vi "20201113_wavelength_measurement_both_wedge_with_DFG_i_it_with_arduino.vi"(0 "Session In":T3) -> (4 "vrt. slope":dbl format="%#_9g", 6 "vert intercept":dbl)   [LabVIEW 2021]
uses:
  <vilib>/userDefined/High Color/IMAQdx.ctl
  <vilib>/Analysis/coordinate.llb/2D Cartesian Coordinate Rotation (Array).vi
  <vilib>/Analysis/6fits.llb/Confidence Interval (Linear).vi
  <vilib>/Instr/_visa.llb/VISA Configure Serial Port (Instr).vi
  <vilib>/Analysis/3filter.llb/Zero Phase Filter (DBL).vi
  <vilib>/addons/control/pid/pid.llb/PID (DBL).vi
  <vilib>/Analysis/3filter.llb/Butterworth Filter (DBL).vi
  <vilib>/Utility/file.llb/Write Delimited Spreadsheet (DBL).vi
  <vilib>/vision/driver/NI_Vision_Acquisition_Software.lvlib
  <vilib>/Analysis/NI_AALPro.lvlib
  <vilib>/Analysis/NI_AAL_SigProc.lvlib
  <vilib>/ptbypt/NI_PtbyPt.lvlib
  <resource>/objmgr/imaqdx.rc
  <vilib>/vision/NI_Vision_Development_Module.lvlib
  <vilib>/Analysis/NI_AALBase.lvlib
  <vilib>/addons/control/pid/NI_PID_pid.lvlib
  <vilib>/LabVIEW Interface for Arduino/LabVIEW Interface for Arduino.lvlib
panel:
  out "number 2":dbl
  out "Boolean":bool
  out "initialized array":dbl[](array[numeric])
  out "subarray 2":dbl[](array[numeric])
  out "Array 5":dbl[](array[numeric])
  out "OPO-532":cluster{dbl[], dbl[]}(graph)
  out "x/y":dbl
  out "cm-1":dbl format="%#_12g"
  out "Amplitudes":dbl[](array[numeric])
  in  "threshold 2":dbl format="%0.2f"
  out "output":dbl format="%.2f"
  out "Vertical intercept vs real time":cluster{dbl[], dbl[]}(graph)
  out "Running average 2":dbl
  out "Running average":dbl
  out "Waveform Graph":dbl[](graph)
  out "Waveform Graph 2":dbl[](graph)
  out "Array 4":dbl[](array[numeric])
  out "loop_counter":i32
  out "vert inteer":dbl[](array[numeric])
  in  "dimension size 2":i32=10
  in  "element 2":dbl=0.1 format="%#_15g"
  in  "Slide 2":dbl(slide)=-10.204081632653061
  out "error out 4":errorcluster
  out "Meter":dbl(knob) scale=0.02..0.1 scale format="%#_4g"
  in  "CONTRAST CUTT OFF VALUE":ext=0.015 format="%#_13g"
  out "x-y":ext
  in  "element":dbl=0.1 format="%#_15g"
  in  "dimension size":i32=10
  out "VERT FRINGE":dbl[][](graph)
  in  "Slide":dbl(slide)=-2.6530612244897958
  out "Verticle slope":cluster{dbl[], dbl[]}(graph)
  out "horz intercept value":dbl[](array[numeric])
  out "vert wavelength":cluster{dbl[], dbl[]}(graph)
  out "intercept":dbl
  in  "index 4":i32=30
  in  "vert-vertical_array length":i32=850
  in  "index 3":i32=500
  in  "length 3":i32=1112
  out "horizontal fringe 2":dbl[][](graph)
  in  "length 2":i32=501
  in  "index 2":i32=400
  in  "length":i32=660
  in  "index":i32=90
  out "vert.wl":dbl
  out "d value":dbl format="%#_10e"
  in  "contrast":ext(slide)=0.5 scale=0.0..0.5 scale format="%#_12g"
  in  "order 2":i32=2
  in  "order":i32=1
  in  "thor wedge spacing":dbl=4.997771500000001 step=1e-06 format="%#_13g"
  in  "wedge angle of thor wedge":dbl=0.004681980000000043 format="%#_13g"
  out "second pass wl 2":dbl format="%#_9g"
  in  "horz. fringe width":i32=6 min=3
  out "hor. std dev":dbl format="%0.5f"
  in  "camera property":bool
  in  "saturation":u32(slide) scale=0.0..128.0
  in  "Gain":u32(slide)=1 scale=1.0..128.0
  in  "exposure":ext(slide)=0.5 scale=0.0..0.5 scale format="%#_12g"
  out "EnumStrings[]":string[](array[string])
  out "known wavelength":dbl
  in  "vert width":i32=5 min=3
  out "Locations":dbl[](array[numeric])
  out "x > y?":bool
  out "Buffer Number Out":u32
  out "observed wavelength":dbl
  out "horz.intercept":dbl format="%#_8g"
  out "known wl":dbl[](array[numeric])=[591.188, 591.588, 591.988, 592.388, 592.788, 593.188]
  out "obseved wl":dbl[](array[numeric])=[591.1849, 591.5523, 591.984, 592.366, 592.7809, 593.169]
  out "standard deviation":dbl format="%0.5f"
  out "Loop time (ms) 2":u32
  out "Array 3":ext[](array[numeric])
  out "Array 2":dbl[](array[numeric])
  out "Array":dbl[](array[numeric])
  out "count":dbl
  out "horz.slope":dbl format="%#_7g"
  out "?":string
  out "?":string
  out "initial time":u32
  out "initial array vert":ext[](array[numeric])
  out "Y Resolution":i32
  out "X Resolution":i32
  out "initial array horz":ext[](array[numeric])
  out "initial array vert.  fringe":ext[](array[numeric])
  out "initila array horz. fringe":ext[](array[numeric])
  in  "Tab Control":enum32{"real time wavelength measurement"}(tab)
  out "532 data":bool
  out "OPO data":bool
  in  "?":T1(tab)
  in  "confidence level vert. fringe":dbl=0.65 format="%.2f"
  in  "threshold vert. fringe":dbl=7.0 format="%0.2f"
  in  "sampling freq. vert. fringe":dbl=1.0000000000000002 format="%0.2f"
  in  "calibration factor vert. fringe":dbl=12000.0
  in  "confidence level horz. fringe":dbl=0.65 format="%.2f"
  in  "sampling freq. horz. fringe":dbl=1.0 format="%0.2f"
  in  "threshold horz. fringe":dbl format="%0.2f"
  in  "calibration factor horz. fringe":dbl=1895.0
  out "RAW Image":T2(plugin-control)
  out "vertical Fringes":dbl[](graph)
  out "Horizontal Fringes":dbl[](graph)
  out "Wavelength vs time":cluster{dbl[], dbl[]}[](graph)
  in  "image depth (bits)":string(combo)="8 bit"
  in  "no. of average":i8=1
  in  "millisecond timer value":u16
  in  "sample length":i32=3
  in  "stop":bool
  in  "Calibration":dbl=7.0
  out "second pass wl":dbl format="%#_9g"
  in  "pixel size (nm)":dbl=4500.0 format="%#_13g"
  in  "wedge angle (rad)":dbl=0.008148144500000017 format="%#_13g"
  in  "wedge spacing":dbl=0.8629192 step=1e-06 format="%#_13g"
  out "?":string="wavelength: 632.993 nm"
  out "?":string
  out "?":string
  in  "maximum OPO":dbl=688.7 format="%#_10g"
  in  "minimum 532":dbl=532.2 format="%#_10g"
  in  "minimum OPO":dbl=688.6 format="%#_10g"
  in  "maximum 532":dbl=532.3 format="%#_10g"
  in  "Running average No":i32=7
  out "Running average OPO data":dbl[](graph)
  out "Running average 532 data":dbl[](graph)
  out "horzontal intercept":cluster{dbl[], dbl[]}(graph)
  out "OPO-532":dbl[](graph)
  in  "Feedback sign":i32=-1 format="%2.0f"
  in  "Manual input voltage":dbl format="%_4f"
  in  "setpoint":dbl format="%.7f"
  in  "output range":cluster{"output high":dbl, "output low":dbl}={"output high"=16.0, "output low"=-16.0} {"output low" format="%.2f"; "output high" format="%.2f"}
  out "Output (V)":dbl format="%.2f"
  in  "PID gains":T4={"proportional gain (Kc)"=1.0, "integral time (Ti, min)"=0.001, "derivative time (Td, min)"=0.001} {"derivative time (Td, min)" format="%.3f"; "integral time (Ti, min)" format="%.3f"; "proportional gain (Kc)" format="%.3f"}
  out "Process value":dbl format="%#_8g"
  in  "Feedback ON":bool
  in  "VISA for power supply 2":refnum<visa-resource-name>
  out "read buffer 2":string
  in  "VISA resource":refnum<visa-resource-name>
  in  "Number Of Servos (1)":u8=1
  in  "DIO Pin (2)":u8=2
  out "Angle (Degrees) 3":u8=15
  in  "millisecond multiple 2":u32=15000
  out "Angle (Degrees)":u8=15
  in  "millisecond multiple":u32=15000
  out "Servo motor Current \nAngle (Degrees) 2":u8=15
  in  "stop 2":bool
  in  "Read voltage":bool
  out "error out 2":errorcluster
  out "error out 3":errorcluster
  out "error out":errorcluster
  # "To do:\n\n(1)  Include calibration routine\n(3) Statistics: Std error for last N values (N is user selected) 1st pass\n-> statistics for deviation of intercept (in cm-1 or MHz) last N values"
  # "Control parameter"
  # "First pass cal."
  # "second pass cal."
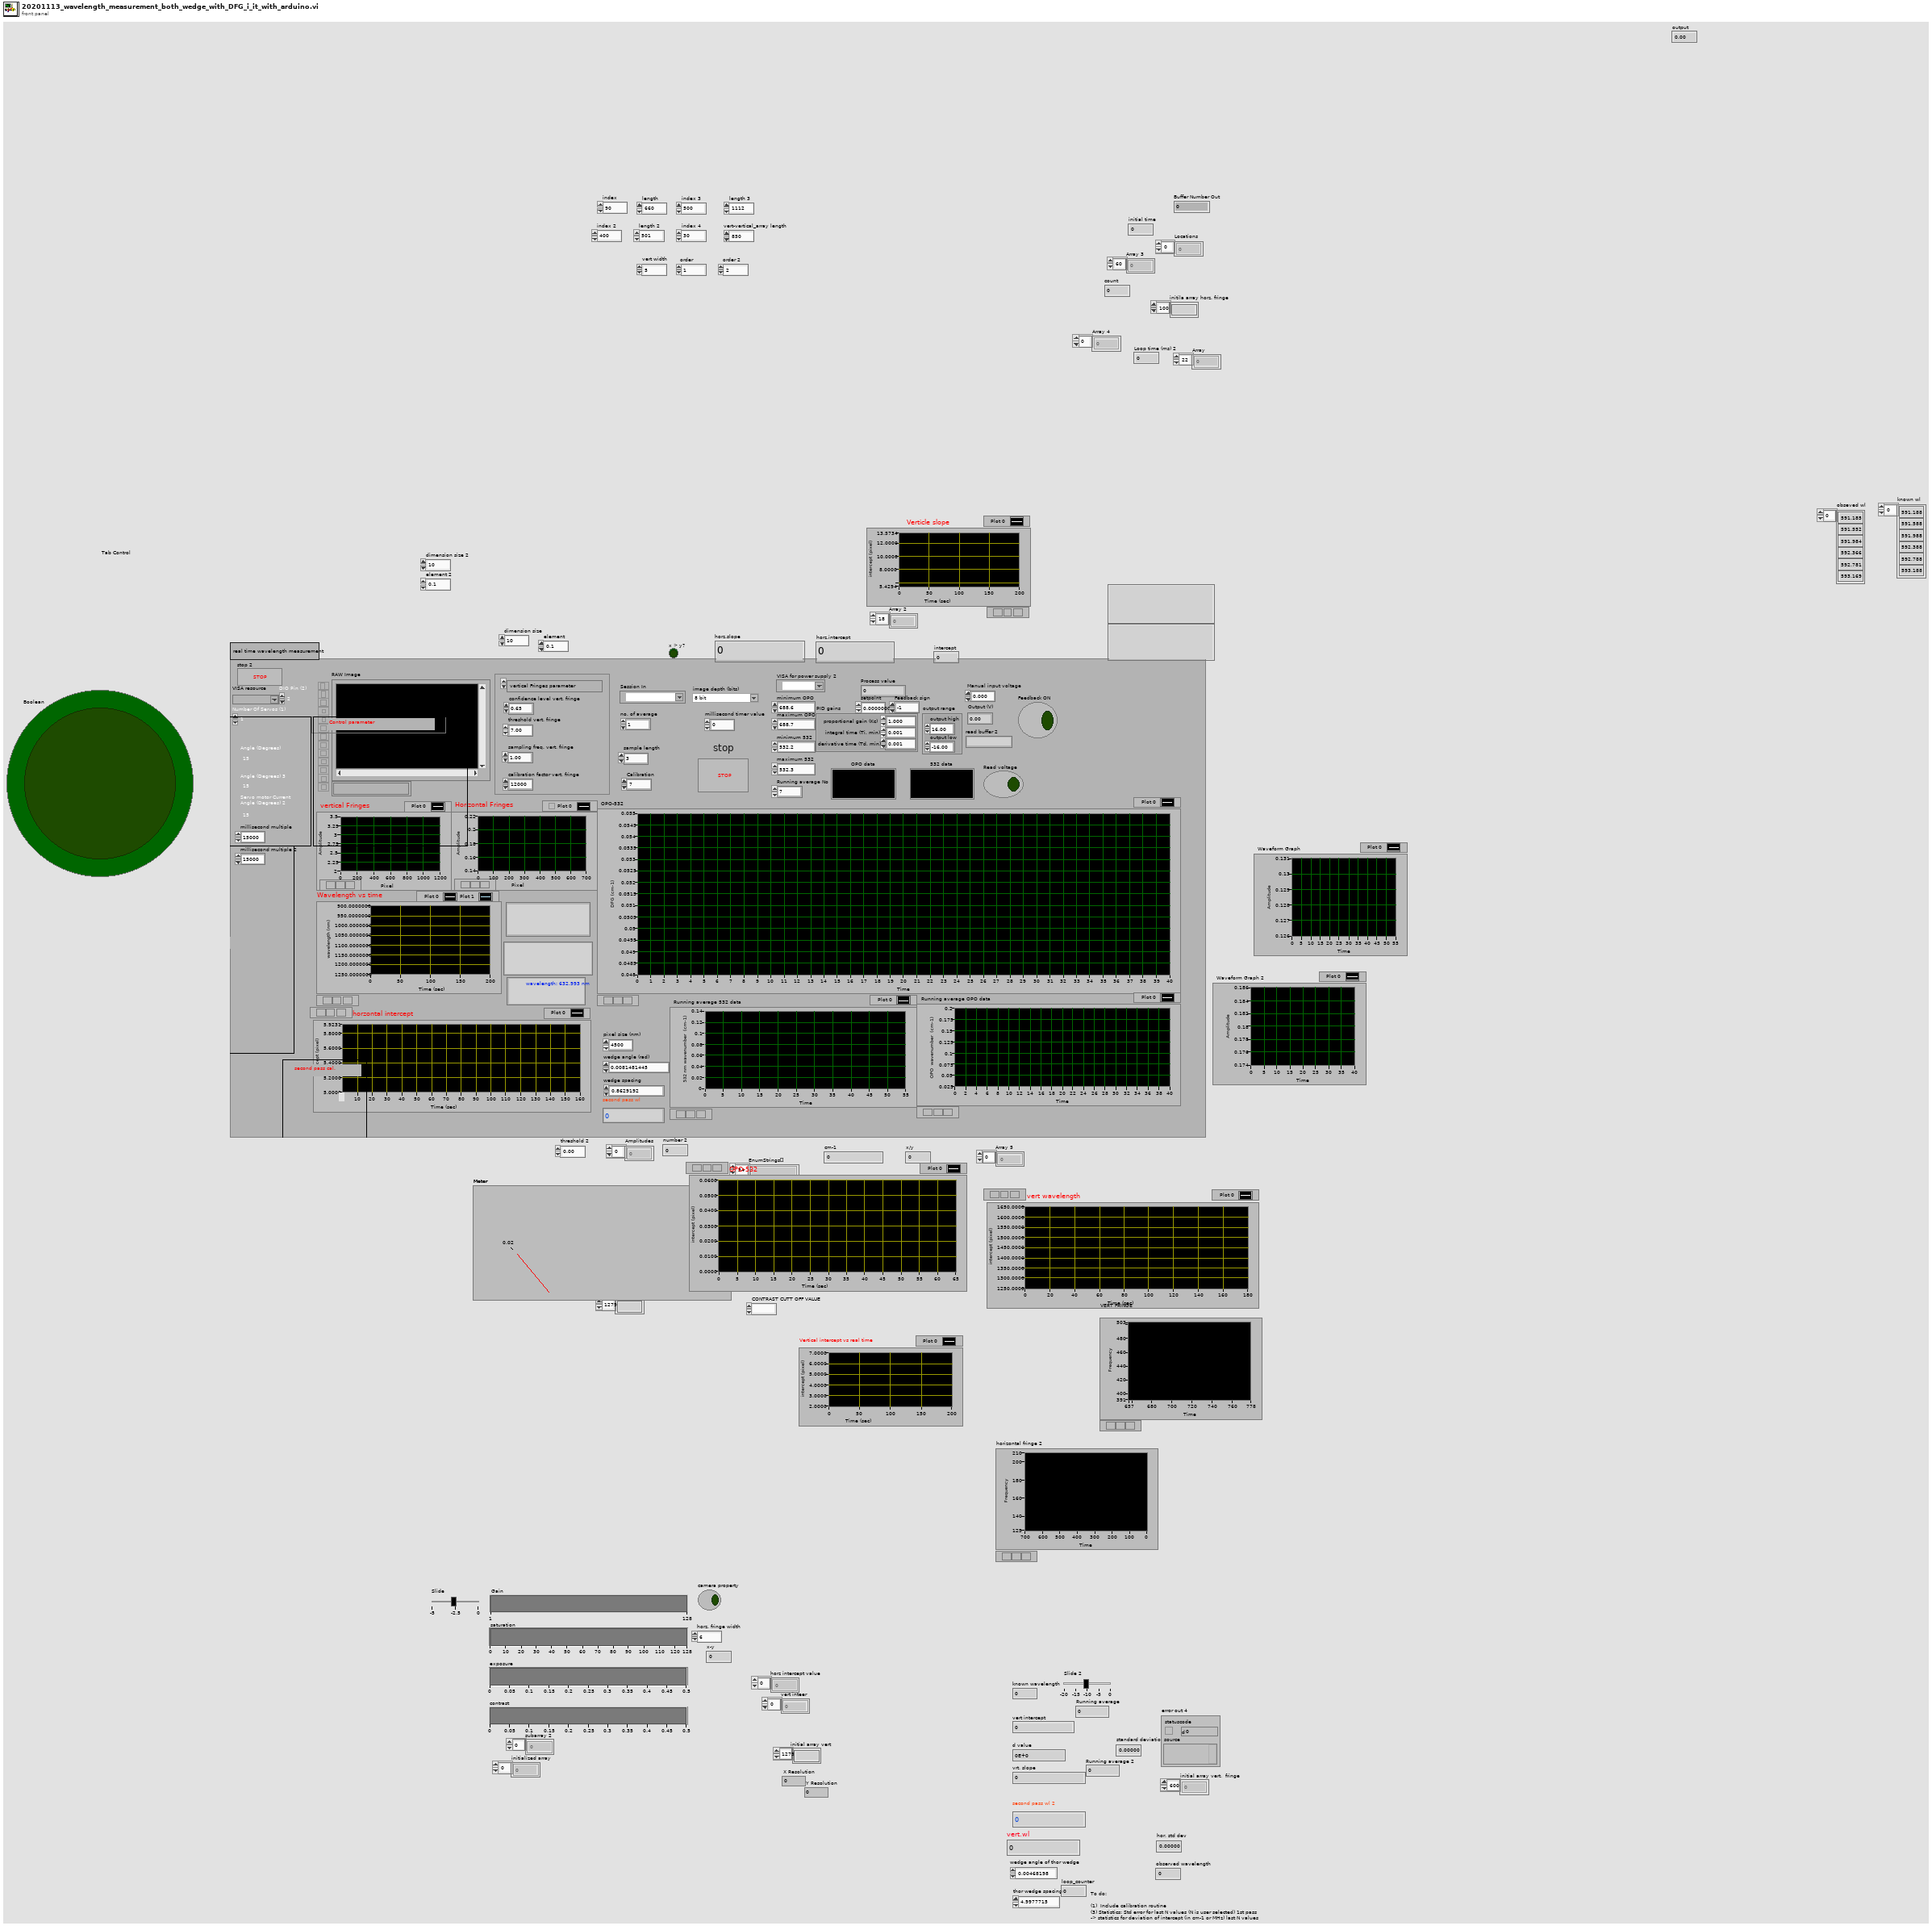
[diagram p1: front panel]
types:
  T1 = enum32{"vertical Fringes parameter", "Horizontal Fringes parameter"}
  T2 = typedef "IMAQ Image.ctl" = refnum<image>
  T3 = typedef "IMAQdx.ctl" = refnum<k21>
  T4 = cluster{"proportional gain (Kc)":dbl, "integral time (Ti, min)":dbl, "derivative time (Td, min)":dbl}
  T5 = typedef "Image Type" = u32
  T6 = typedef "LabVIEW Interface for Arduino.lvlib/Arduino Resource.ctl" = cluster{"VISA resource":refnum<visa-resource-name>, "Board Type":T7, "Connection Type":enum8{"USB / Serial"}, "Bytes Per Packet (15)":u8}
  T7 = typedef "LabVIEW Interface for Arduino.lvlib/Board Type.ctl" = enum16{"Uno", "Dimuelanove w/Atmega 328", "Mega 2560"}
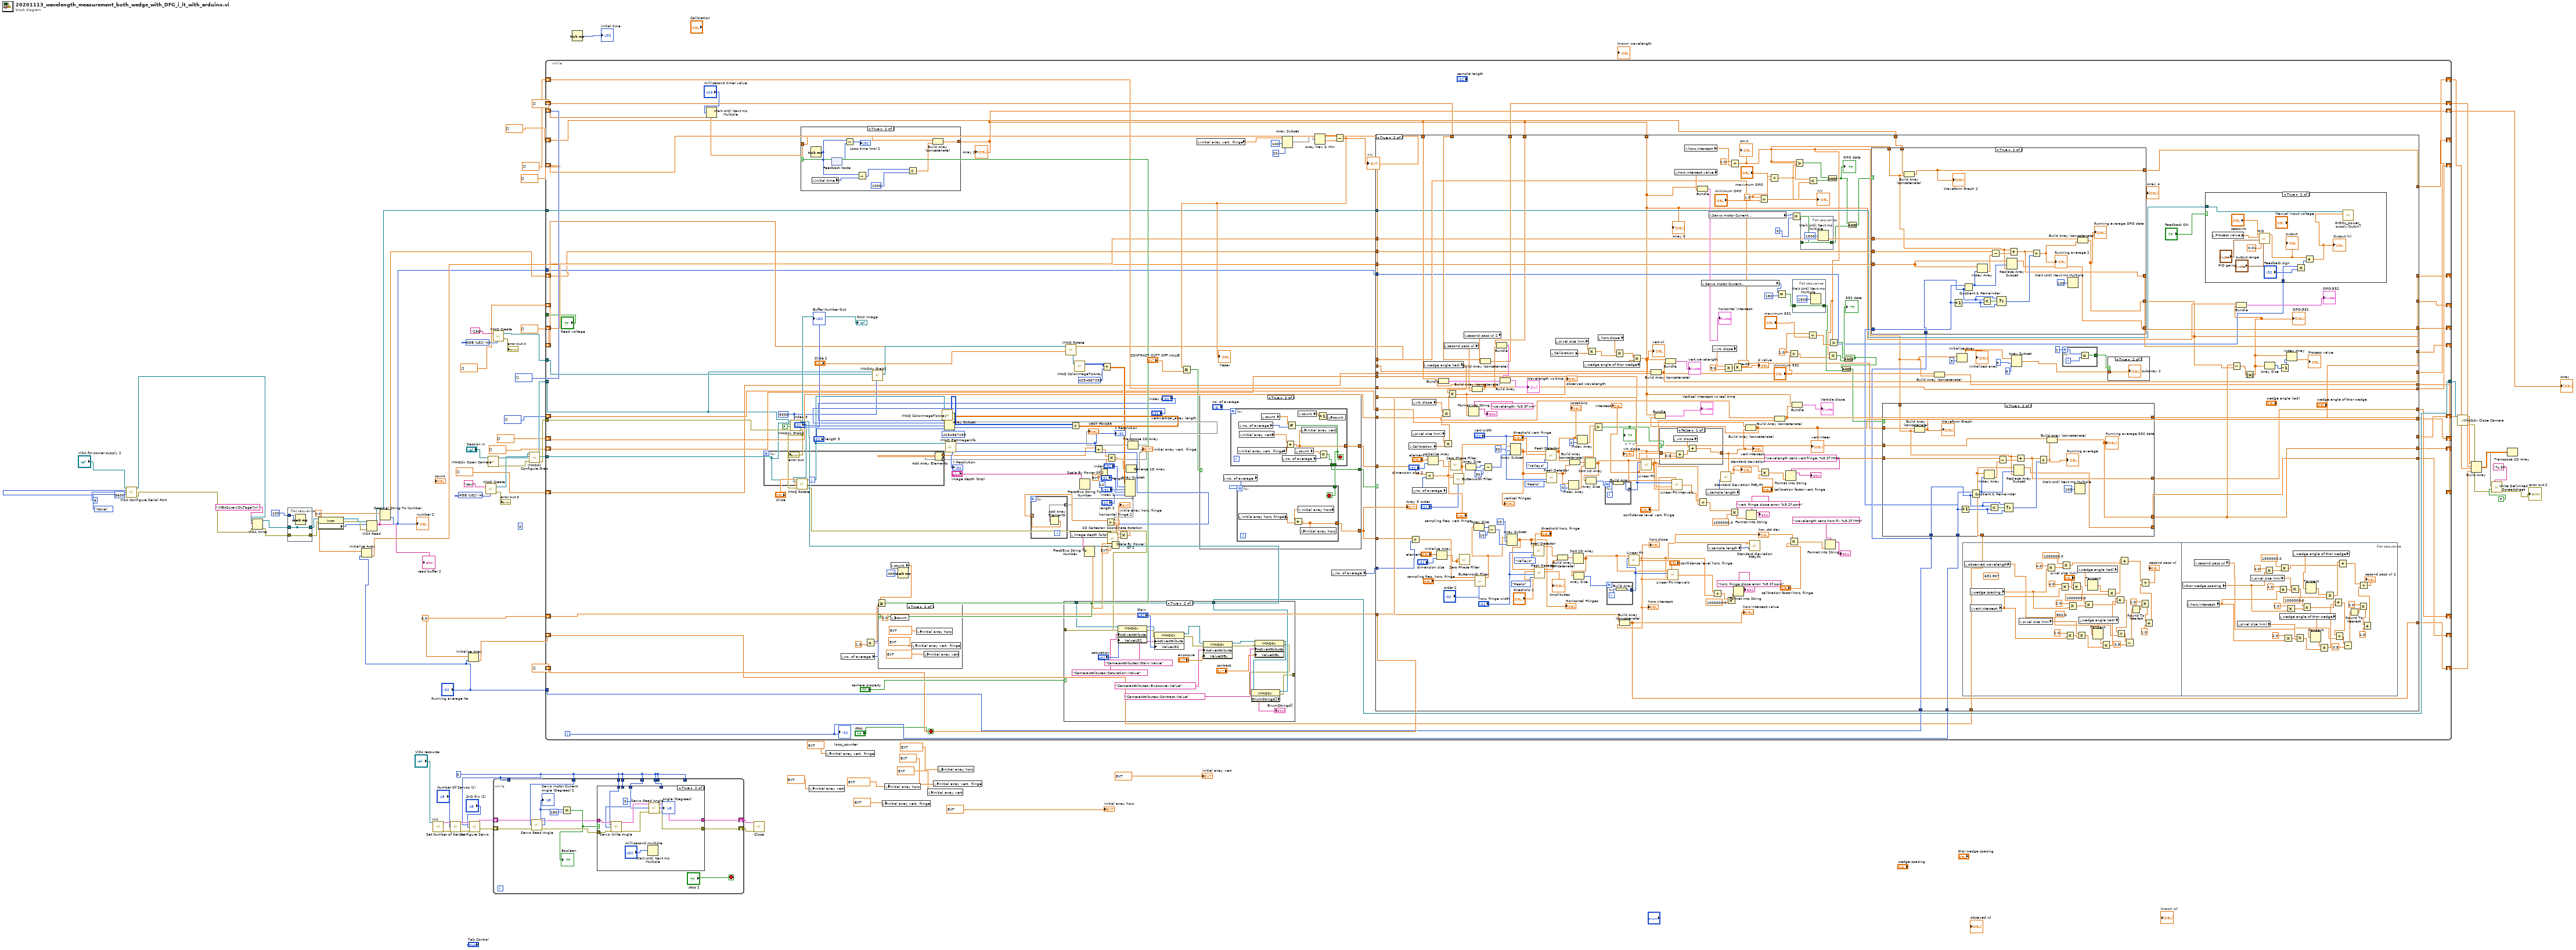
[diagram p0: block diagram]
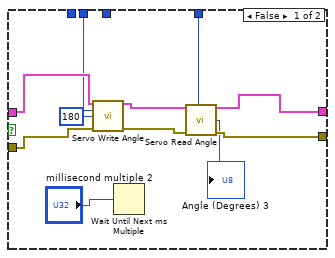
[diagram p2: hidden frame]
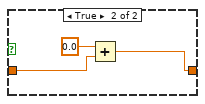
[diagram p12: hidden frame]
diagram:
  w15 = u8 0 ("Servo Number (0)")
  (unwired) u8 0 ("Servo Number (0)")
  w32 = 0.0
  w37 = 0.0
  w54 = T5 4 items=["Grayscale (U8)", "Grayscale (I16)", "Grayscale (SGL)", "Complex (CSG)", "RGB (U32)", "HSL (U32)", "RGB (U64)", "Grayscale (U16)"] ("Image Type")
  w78 = T5 4 items=["Grayscale (U8)", "Grayscale (I16)", "Grayscale (SGL)", "Complex (CSG)", "RGB (U32)", "HSL (U32)", "RGB (U64)", "Grayscale (U16)"] ("Image Type")
  n1 = call-poly "VISA Configure Serial Port"("VISA resource name"="VISA for power supply 2", "baud rate (9600)"=u32 9600, "data bits (8)"=u16 8, "parity (0:none)"=enum16{"None", "Odd", "Even", "Mark", "Space"}."None") -> ("VISA resource name out"=w13:refnum<visa-resource-name>, "error out"=w14:errorcluster)  [unwired: 5 in, 5 out]
  n2 = VISA Write(VISA resource name=w13, write buffer=":MEASure:VOLTage?\n" ("Command"), error in (no error)=w14) -> (VISA resource name out=w11:refnum<visa-resource-name>, error out=w10:errorcluster)  [unwired: 1 out]
  n3 = flat-sequence {
    tunnel: w10 -> [w84]
    tunnel: [w84] -> w8
    tunnel: w11 -> [w83]
    tunnel: [w83] -> _
    tunnel: u32 100 ("delay before read (ms)") -> [w85]
    tunnel: [w83] -> w9
    frame #0 {
      n4 = Wait (ms)(milliseconds to wait=w85) -> ()  [unwired: 1 out]
    }
  }
  n5 = property class="Instr"(reference=w9, error in=w8) -> (reference out=w7:refnum<visa-resource-name>, error out=w6:errorcluster, "Serial Settings:Number of Bytes at Serial Port"=w1:u32)
  n6 = Initialize Array(w32, "Running average No") -> (w33:dbl[])
  n7 = VISA Read(VISA resource name=w7, byte count=w1, error in (no error)=w6) -> (VISA resource name out=w2:refnum<visa-resource-name>, read buffer=w3:string)  [unwired: 2 out]
  "read buffer 2" <- w3
  n8 = Decimal String To Number(string=w3) -> (number=w5:i32)  [unwired: 2 in, 1 out]
  "number 2" <- w5
  n9 = call <vilib>:"Init.vi"("VISA resource"="VISA resource") -> ("Arduino Resource"=w26:T6, "error out"=w25:errorcluster)  [unwired: 17 in]
  n10 = call <vilib>:"Set Number of Servos.vi"("Arduino Resource"=w26, "Number Of Servos (1)"="Number Of Servos (1)", "error in"=w25) -> ("Arduino Resource"=w21:T6, "error out"=w20:errorcluster)  [unwired: 11 in]
  n11 = Initialize Array(w37, "Running average No") -> (w38:dbl[])
  n12 = call <vilib>:"Configure Servo.vi"("Arduino Resource"=w21, "Servo Number (0)"=w15, "DIO Pin (2)"="DIO Pin (2)", "error in"=w20) -> ("Arduino Resource"=w19:T6, "error out"=w18:errorcluster)  [unwired: 10 in]
  n13 = call "IMAQ Create"("Image Name"="sau", "Image Type"=w78) -> ("New Image"=w76:T2, "error out"=→"error out 3":errorcluster)  [unwired: 3 in]
  n14 = call <vilib>:"IMAQdx Open Camera.vi"("Session In"="Session In") -> ("error out"=w56:errorcluster, "Session Out"=w55:T3)  [unwired: 9 in]
  n15 = call "IMAQ Create"("Image Name"="256", "Image Type"=w54) -> ("New Image"=w51:T2, "error out"=→"error out 4":errorcluster)  [unwired: 3 in]
  n16 = while {
    tunnel: w15 -> [w100]
    shift-right: [w94] -> w24
    shift-left: w19 -> [w89]
    shift-right: [w93] -> w23
    shift-left: w18 -> [w88]
    tunnel: w15 -> [_]
    tunnel: w15 -> [_]
    tunnel: w15 -> [w95]
    tunnel: w15 -> [_]
    tunnel: w15 -> [w92]
    tunnel: w15 -> [w91]
    tunnel: w15 -> [w90]
    stop <- "stop 2" stop-if-true
    n17 = call <vilib>:"Servo Read Angle.vi"("Arduino Resource"=w89, "Servo Number"=w100, "error in"=w88) -> ("Arduino Resource"=w97:T6, "Angle (Degrees)"=w99:u8, "error out"=w96:errorcluster)  [unwired: 10 in]
    "Servo motor Current \nAngle (Degrees) 2" <- w99
    n18 = Equal?(x=w99, y=u8 180) -> (x = y?=w87:bool)
    "Boolean" <- w87
    n19 = case shown="True" w87 {
      tunnel: w97 -> [w109 w122]
      tunnel: w96 -> [w108 w121]
      tunnel: w95 -> [_ w120]
      tunnel: [w105 w114] -> w94
      tunnel: [w106 w116] -> w93
      tunnel: w92 -> [_ w113]
      tunnel: w91 -> [w104 _]
      tunnel: w90 -> [w103 _]
      frame False {
        n20 = call <vilib>:"Servo Write Angle.vi"("Arduino Resource"=w109, "Servo Number"=w104, "Angle (Degrees)"=u8 180, "error in"=w108) -> ("Arduino Resource"=w110:T6, "error out"=w107:errorcluster)  [unwired: 10 in]
        n21 = Wait Until Next ms Multiple(millisecond multiple="millisecond multiple 2") -> ()  [unwired: 1 out]
        n22 = call <vilib>:"Servo Read Angle.vi"("Arduino Resource"=w110, "Servo Number"=w103, "error in"=w107) -> ("Arduino Resource"=w105:T6, "Angle (Degrees)"=→"Angle (Degrees) 3":u8, "error out"=w106:errorcluster)  [unwired: 10 in]
      }
      frame True {
        n23 = call <vilib>:"Servo Write Angle.vi"("Arduino Resource"=w122, "Servo Number"=w120, "Angle (Degrees)"=u8 0, "error in"=w121) -> ("Arduino Resource"=w115:T6, "error out"=w117:errorcluster)  [unwired: 10 in]
        n24 = Wait Until Next ms Multiple(millisecond multiple="millisecond multiple") -> ()  [unwired: 1 out]
        n25 = call <vilib>:"Servo Read Angle.vi"("Arduino Resource"=w115, "Servo Number"=w113, "error in"=w117) -> ("Arduino Resource"=w114:T6, "Angle (Degrees)"=→"Angle (Degrees)":u8, "error out"=w116:errorcluster)  [unwired: 10 in]
      }
    }
  }
  n26 = call <vilib>:"IMAQdx Configure Grab.vi"("error in"=w56, "Session In"=w55) -> ("error out"=w75:errorcluster, "Session Out"=w81:T3)  [unwired: 8 in]
  n27 = while {
    tunnel: w75 -> [w232]
    tunnel: w76 -> [w167]
    tunnel: w81 -> [w127]
    tunnel: [w201] -> w72
    shift-right: [w203] -> w48
    shift-left: i32[] [] -> [w225]
    shift-right: [w210] -> w41
    shift-left: dbl[] [] -> [w205]
    shift-right: [w197] -> w61
    shift-left: u32[] [] -> [w211]
    shift-right: [w198] -> w47
    shift-left: dbl[] [] -> [w199]
    shift-right: [w186] -> w46
    shift-left: dbl[] [] -> [w185]
    shift-right: [w183] -> _
    shift-left: dbl[] [] -> [w182]
    shift-right: [w150] -> _
    shift-left: dbl[] [] -> [w179]
    tunnel: w51 -> [w128]
    shift-right: [w148] -> _
    shift-left: dbl[] [] -> [w147]
    shift-right: [w146] -> _
    shift-left: dbl[] [] -> [w145]
    tunnel: "Running average No" -> [w143]
    shift-right: [w142] -> _
    shift-left: w38 -> [w141]
    shift-right: [w140] -> _
    shift-left: w37 -> [w139]
    shift-right: [w137] -> _
    shift-left: dbl[] [] -> [w138]
    shift-right: [w133] -> _
    shift-left: dbl[] [] -> [w136]
    shift-right: [w135] -> _
    shift-left: w33 -> [w134]
    shift-right: [w132] -> _
    shift-left: w32 -> [w131]
    shift-right: [w130] -> _
    shift-left: dbl[] [] -> [w129]
    tunnel: ["Read voltage"] -> _
    tunnel: w5 -> [w124]
    tunnel: w2 -> [w123]
    i -> [w144]
    stop <- "stop" stop-if-true
    w157 = 5000 ("Timeout (ms)")
    n28 = Wait Until Next ms Multiple(millisecond multiple="millisecond timer value") -> ()  [unwired: 1 out]
    n29 = call <vilib>:"IMAQdx Grab2.vi"("Timeout (ms)"=w157, "error in"=w232, "Wait for Next Buffer? (Yes)"=FALSE, "Image In"=w167, "Session In"=w127) -> ("error out"=w170:errorcluster, "Buffer Number Out"=→"Buffer Number Out":u32, "Image Out"=w168:T2, "Session Out"=w202:T3)  [unwired: 3 in]
    "error out" <- w170
    "RAW Image" <- w168
    n30 = call "IMAQ Rotate"("error in (no error)"=w170, "Angle (degrees)"="Slide", "Image Dst"=w168, "Image Src"=w167) -> ("error out"=w169:errorcluster, "Image Dst Out"=w171:T2)  [unwired: 6 in]
    n31 = local read "no. of average"() -> (w214:i8)
    n32 = Add(x=w214, y=1.0) -> (x+y=w213:dbl)
    n33 = call <vilib>:"IMAQdx Grab2.vi"("Timeout (ms)"=w157, "Image In"=w128, "Session In"=w127) -> ("Image Out"=w152:T2)  [unwired: 5 in, 3 out]
    n34 = local read "count"() -> (w216:dbl)
    n35 = Greater Or Equal?(x=w216, y=w213) -> (x >= y?=w212:bool)
    n36 = case shown="True" w212 {
      tunnel: [w277 w280] -> w197
      tunnel: w211 -> [w277 w278]
      frame False {
      }
      frame True {
        n37 = Tick Count (ms)() -> (millisecond timer value=w281:u32)
        n38 = local read "initial time"() -> (w285:u32)
        n39 = feedback #1() -> (w286:u32)  [unwired: 1 in]
        n40 = feedback-in #1(w281) -> ()
        n41 = Subtract(x=w281, y=w286) -> (x-y=→"Loop time (ms) 2":u32)
        n42 = Subtract(x=w281, y=w285) -> (x-y=w282:u32)
        n43 = Divide(x=w282, y=1000) -> (x/y=w279:dbl)
        n44 = Build Array (concatenate)(w278, w279) -> (w280:dbl[])
      }
    }
    "Array 2" <- w197
    n45 = case shown="True" w212 {
      frame False {
      }
      frame True {
        n46 = local write "count"(0.0 ("count")) -> ()
        n47 = local write "initial array vert.  fringe"(ext[] array[1280 elements] ("initial array")) -> ()
        n48 = local write "initial array horz"(ext[] array[1280 elements] ("initial array 2")) -> ()
        n49 = local write "initial array vert"(ext[] array[1282 elements] ("initial array vert")) -> ()
      }
    }
    n50 = Wait (ms)(milliseconds to wait=u32 400) -> ()  [unwired: 1 out]
    n51 = call "IMAQ ColorImageToArray"("Image"=w171) -> ("Image Pixels (U32)"=w229:u32[][])  [unwired: 3 in, 2 out]
    n52 = call "IMAQ GetImageInfo"("Image"=w171) -> ("Y Resolution"=w227:i32, "X Resolution"=w226:i32)  [unwired: 3 in, 6 out]
    "Y Resolution" <- w227
    "X Resolution" <- w226
    n53 = case shown="True" "camera property" {
      tunnel: w169 -> [w254 w256]
      tunnel: w202 -> [w255 w257]
      tunnel: [w255 w266] -> w201
      tunnel: [w254 w264] -> _
      frame False {
      }
      frame True {
        n54 = property class="IMAQdx"(reference=w257, error in=w256, "ActiveAttribute"="CameraAttributes::Saturation::Value", "ValueU32"="saturation") -> (reference out=w269:T3, error out=w270:errorcluster)
        n55 = property class="IMAQdx"(reference=w269, error in=w270, "ActiveAttribute"="CameraAttributes::Gain::Value", "ValueU32"="Gain") -> (reference out=w274:T3, error out=w273:errorcluster)
        n56 = property class="IMAQdx"(reference=w274, error in=w273, "ActiveAttribute"="CameraAttributes::Exposure::Value", "ValueDBL"="exposure") -> (reference out=w263:T3, error out=w259:errorcluster)
        n57 = property class="IMAQdx"(reference=w263, error in=w259, "ActiveAttribute"="CameraAttributes::Contrast::Value", "ValueDBL"="contrast") -> (reference out=w262:T3, error out=w258:errorcluster)
        n58 = property class="IMAQdx"(reference=w262, error in=w258) -> (reference out=w266:T3, error out=w264:errorcluster, "EnumStrings[]"=→"EnumStrings[]":string[])
      }
    }
    n59 = call "IMAQ Rotate"("Angle (degrees)"="Slide 2", "Image Src"=w152) -> ("Image Dst Out"=w151:T2)  [unwired: 8 in, 1 out]
    n60 = Divide(x=w229, y=u32 4294967295) -> (x/y=w180:dbl[][])
    n61 = Array Subset(array=w180, index (row)="index 4", length (row)="vert-vertical_array length", index (col)="index 3", length (col)="length 3") -> (w188:dbl[][])
    n62 = local read "image depth (bits)"() -> (w206:string)
    n63 = call "IMAQ ColorImageToArray"("Image"=w151) -> ("Image Pixels (U32)"=w156:u32[][])  [unwired: 3 in, 2 out]
    n64 = Fract/Exp String To Number(string="image depth (bits)") -> ()  [unwired: 3 in, 2 out]
    n65 = Fract/Exp String To Number(string=w206) -> (number=w207:dbl)  [unwired: 3 in, 1 out]
    n66 = Scale By Power Of 2(n=i16 12, x=ext 1.0) -> (x*2^n=w221:ext)
    n67 = Divide(x=w156, y=u32 4294967295) -> (x/y=w154:dbl[][])
    n68 = call-poly <vilib>:"2D Cartesian Coordinate Rotation.vi"() -> ()  [unwired: 9 in, 3 out]
    n69 = Scale By Power Of 2(n=w207, x=ext 1.0) -> (x*2^n=w217:ext)
    n70 = Array Subset(array=w154, index (row)="index", length (row)="length", index (col)="index 2", length (col)="length 2") -> (w193:dbl[][])
    "horizontal fringe 2" <- w193
    n71 = for {
      tunnel: [w653] -> w220 mode=indexing
      tunnel: w193 -> [w652] mode=indexing
      n72 = Add Array Elements(numeric array=w652) -> (sum=w653:dbl)
    }
    n73 = Divide(x=w220, y=w226) -> (x/y=w219:dbl[])
    n74 = Multiply(x=w219, y=w217) -> (x*y=→"initila array horz. fringe":ext[])
    n75 = Transpose 2D Array(2D array=w188) -> (transposed array=w166:dbl[][])
    "VERT FRINGE" <- w166
    n76 = for {
      tunnel: [w655] -> w224 mode=indexing
      tunnel: w166 -> [w654] mode=indexing
      n77 = Add Array Elements(numeric array=w654) -> (sum=w655:dbl)
    }
    n78 = Divide(x=w224, y=w227) -> (x/y=w223:dbl[])
    n79 = Multiply(x=w223, y=w221) -> (x*y=w187:ext[])
    n80 = Reverse 1D Array(array=w187) -> (reversed array=→"initial array vert.  fringe":ext[])
    n81 = local read "initial array vert.  fringe"() -> (w164:ext[])
    n82 = Array Subset(array=w164, index=100, length=20) -> (w163:ext[])
    n83 = Array Max & Min(array=w163) -> (max value=w162:ext, min value=w161:ext)  [unwired: 2 out]
    n84 = local read "no. of average"() -> (w209:i8)
    n85 = Subtract(x=w162, y=w161) -> (x-y=w158:ext)
    "x-y" <- w158
    "Meter" <- w158
    n86 = Greater Or Equal?(x=w158, y="CONTRAST CUTT OFF VALUE") -> (x >= y?=w160:bool)
    n87 = case shown="True" w160 {
      tunnel: [_ w235] -> w177
      tunnel: [_ w234] -> w175
      tunnel: [_ w233] -> w165
      frame False {
      }
      frame True {
        n88 = local read "no. of average"() -> (w237:i8)
        n89 = for {
          N: "no. of average" -> [_]
          tunnel: [w251] -> w235
          tunnel: [w246] -> w233
          tunnel: [w243] -> w236
          stop <- w243 stop-if-true
          n90 = local read "initial array vert.  fringe"() -> (w253:ext[])
          n91 = local read "no. of average"() -> (w244:i8)
          n92 = local read "initial array vert"() -> (w252:ext[])
          n93 = local read "count"() -> (w245:dbl)
          n94 = local read "no. of average"() -> (w250:i8)
          n95 = Add(x=w252, y=w253) -> (x+y=w251:ext[])
          n96 = Not Equal?(x=w245, y=w244) -> (x != y?=w243:bool)
          n97 = local read "count"() -> (w249:dbl)
          n98 = local read "count"() -> (w248:dbl)
          n99 = local write "initial array vert"(w251) -> ()
          n100 = Increment(x=w248) -> (x+1=w247:dbl)
          n101 = Equal?(x=w249, y=w250) -> (x = y?=w246:bool)
          n102 = local write "count"(w247) -> ()
        }
        n103 = for {
          N: w237 -> [_]
          tunnel: [w242] -> w234
          tunnel: w236 -> [w239]
          stop <- w239 stop-if-true
          n104 = local read "initila array horz. fringe"() -> (w240:ext[])
          n105 = local read "initial array horz"() -> (w241:ext[])
          n106 = Add(x=w241, y=w240) -> (x+y=w242:ext[])
          n107 = local write "initial array horz"(w242) -> ()
        }
      }
    }
    "Array 3" <- w175
    n108 = case shown="True" w165 {
      tunnel: [w304 w475] -> w203
      tunnel: w225 -> [w304 w502]
      tunnel: w175 -> [_ w500]
      tunnel: w177 -> [_ w499]
      tunnel: w197 -> [_ w480]
      tunnel: [w305 w330] -> w210
      tunnel: w197 -> [_ w332]
      tunnel: w209 -> [_ w479]
      tunnel: w205 -> [w305 w476]
      tunnel: [w303 w421] -> w198
      tunnel: w199 -> [w303 w423]
      tunnel: w197 -> [_ w422]
      tunnel: [w302 w399] -> w186
      tunnel: w185 -> [w302 w400]
      tunnel: w182 -> [w301 w397]
      tunnel: [w301 w396] -> w183
      tunnel: w179 -> [w300 w393]
      tunnel: [w300 w390] -> w150
      tunnel: w147 -> [w299 w373]
      tunnel: [w299 w374] -> w148
      tunnel: [w298 w367] -> w146
      tunnel: w145 -> [w298 w368]
      tunnel: w144 -> [_ w358]
      tunnel: w143 -> [_ w359]
      tunnel: w141 -> [w297 w366]
      tunnel: [w297 w365] -> w142
      tunnel: [w296 w364] -> w140
      tunnel: w139 -> [w296 w363]
      tunnel: w138 -> [w295 w362]
      tunnel: [w295 w333] -> w137
      tunnel: w136 -> [w293 w361]
      tunnel: w134 -> [w294 w360]
      tunnel: [w294 w357] -> w135
      tunnel: [w293 w334] -> w133
      tunnel: w131 -> [w292 w356]
      tunnel: [w292 w355] -> w132
      tunnel: w123 -> [_ w353]
      tunnel: w124 -> [_ w352]
      tunnel: w129 -> [w291 w329]
      tunnel: [w291 w321] -> w130
      frame False {
      }
      frame True {
        w337 = 1.0 ("x")
        w342 = 1.0 ("x")
        n109 = local read "Calibration"() -> (w442:dbl)
        n110 = Divide(x=w500, y=w479) -> (x/y=w381:ext[])
        n111 = local read "pixel size (nm)"() -> (w440:dbl)
        n112 = local read "vrt. slope"() -> (w447:dbl)
        n113 = local read "no. of average"() -> (w501:i8)
        n114 = local read "wedge angle (rad)"() -> (w443:dbl)
        n115 = Divide(x=w499, y=w501) -> (x/y=w384:ext[])
        n116 = Initialize Array("element 2", "dimension size 2") -> (w387:dbl[])
        n117 = Initialize Array("element", "dimension size") -> (w383:dbl[])
        n118 = Multiply(x=w440, y=w442) -> (x*y=w441:dbl)
        n119 = Multiply(x=w447, y=w441) -> (x*y=w446:dbl)
        n120 = local read "second pass wl"() -> (w445:dbl)
        n121 = Multiply(x=w443, y=w446) -> (x*y=w444:dbl)
        "observed wavelength" <- w444
        n122 = call-poly <vilib>:"Zero Phase Filter.vi"("Forward Coefficients"=w387, "X"=w384) -> ()  [unwired: 8 in, 2 out]
        n123 = call-poly <vilib>:"Butterworth Filter.vi"("order"="order", "sampling freq: fs"="sampling freq. vert. fringe", "X"=w384) -> ("Filtered X"=w382:dbl[])  [unwired: 5 in, 1 out]
        n124 = call-poly <vilib>:"Zero Phase Filter.vi"("Forward Coefficients"=w383, "Reverse Coefficients"=w383) -> ()  [unwired: 8 in, 2 out]
        n125 = local read "second pass wl 2"() -> (w424:dbl)
        n126 = Array Size(array=w382) -> (size(s)=w428:i32)
        n127 = Format Into String(format string="wavelength: %5.3f nm", w444) -> (resulting string=→"?":string)  [unwired: 2 in, 1 out]
        n128 = Build Array (concatenate)(w476, w445) -> (w330:dbl[])
        n129 = Bundle(w480, w330) -> (w419:cluster{dbl[], dbl[]})  [unwired: 1 in]
        n130 = call-poly <vilib>:"Butterworth Filter.vi"("order"="order 2", "sampling freq: fs"="sampling freq. horz. fringe", "X"=w381) -> ("Filtered X"=w380:dbl[])  [unwired: 5 in, 1 out]
        n131 = Array Size(array=w380) -> (size(s)=w431:i32)
        n132 = Build Array (concatenate)(w423, w424) -> (w421:dbl[])
        n133 = Subtract(x=w428, y=50) -> (x-y=w426:i32)
        n134 = Subtract(x=w431, y=10) -> (x-y=w430:i32)
        n135 = Bundle(w422, w330) -> (w420:cluster{dbl[], dbl[]})  [unwired: 1 in]
        n136 = Build Array(w420, w419) -> (→"Wavelength vs time":cluster{dbl[], dbl[]}[])
        n137 = Array Subset(array=w380, index=10, length=w430) -> (w412:dbl[])
        "Horizontal Fringes" <- w412
        n138 = Array Subset(array=w382, index=30, length=w426) -> (w402:dbl[])
        "vertical Fringes" <- w402
        n139 = call <vilib>:"Peak Detector.vi"("peaks/valleys"=enum32{"Peaks", "Valleys"}."Valleys", "width"="horz. fringe width", "threshold"="threshold horz. fringe", "X"=w412) -> ("Locations"=w471:dbl[])  [unwired: 3 in, 4 out]
        n140 = call <vilib>:"Peak Detector.vi"("peaks/valleys"=enum32{"Peaks", "Valleys"}."Peaks", "width"="horz. fringe width", "threshold"="threshold 2", "X"=w412) -> ("Amplitudes"=→"Amplitudes":dbl[], "Locations"=w470:dbl[])  [unwired: 3 in, 3 out]
        n141 = call <vilib>:"Peak Detector.vi"("peaks/valleys"=enum32{"Peaks", "Valleys"}."Valleys", "width"="vert width", "threshold"="threshold vert. fringe", "X"=w402) -> ("Locations"=w457:dbl[])  [unwired: 3 in, 4 out]
        "Locations" <- w457
        n142 = call <vilib>:"Peak Detector.vi"("peaks/valleys"=enum32{"Peaks", "Valleys"}."Peaks", "width"="vert width", "X"=w402) -> ("Locations"=w450:dbl[])  [unwired: 4 in, 4 out]
        n143 = local read "Calibration"() -> (w408:dbl)
        n144 = local read "pixel size (nm)"() -> (w409:dbl)
        n145 = Build Array (concatenate)(w471, w470) -> (w469:dbl[])
        n146 = Index Array(array=w450, index=0) -> (element=w453:dbl)
        n147 = Build Array (concatenate)(w457, w450) -> (w495:dbl[])
        n148 = Sort 1D Array(array=w469) -> (sorted array=w466:dbl[])
        n149 = Array Size(array=w466) -> (size(s)=w468:i32)
        n150 = Index Array(array=w457, index=0) -> (element=w454:dbl)
        n151 = local read "wedge angle of thor wedge"() -> (w404:dbl)
        n152 = Sort 1D Array(array=w495) -> (sorted array=w493:dbl[])
        n153 = Array Size(array=w493) -> (size(s)=w494:i32)
        n154 = Multiply(x=w409, y=w408) -> (x*y=w406:dbl)
        n155 = Greater?(x=w454, y=w453) -> (0:w452:bool)
        "x > y?" <- w452
        n156 = local read "horz.slope"() -> (w407:dbl)
        n157 = for {
          N: w494 -> [_]
          tunnel: [w651] -> w492 mode=concatenating
          i -> [w650]
          n158 = Build Array(w650) -> (w651:i32[])
        }
        n159 = for {
          N: w468 -> [_]
          tunnel: [w577] -> w467 mode=concatenating
          i -> [w576]
          n160 = Build Array(w576) -> (w577:i32[])
        }
        n161 = Multiply(x=w407, y=w406) -> (x*y=w405:dbl)
        n162 = call <vilib>:"Linear Fit.vi"("Y"=w466, "X"=w467) -> ("slope"=w462:dbl, "intercept"=w401:dbl)  [unwired: 9 in, 3 out]
        "horz.slope" <- w462
        "horz.intercept" <- w401
        n163 = Build Array (concatenate)(w400, w401) -> (w399:dbl[])
        "horz intercept value" <- w399
        n164 = Multiply(x=w405, y=w404) -> (x*y=w398:dbl)
        "vert.wl" <- w398
        n165 = call <vilib>:"Linear Fit.vi"("Y"=w493, "X"=w492) -> ("slope"=w392:dbl, "intercept"=w458:dbl)  [unwired: 9 in, 3 out]
        "vrt. slope" <- w392
        "intercept" <- w458
        n166 = Build Array (concatenate)(w397, w398) -> (w396:dbl[])
        n167 = case shown="False" w452 {
          tunnel: w458 -> [w570 w575]
          tunnel: [w572 w574] -> w403
          frame False {
            n168 = local read "vrt. slope"() -> (w571:dbl)
            n169 = Add(x=w570, y=0.0) -> (x+y=w569:dbl)
            n170 = Add(x=w571, y=w569) -> (x+y=w572:dbl)
          }
          frame True {
            n171 = Add(x=0.0, y=w575) -> (x+y=w574:dbl)
          }
        }
        "vert intercept" <- w403
        n172 = Bundle(w332, w396) -> (→"vert wavelength":cluster{dbl[], dbl[]})  [unwired: 1 in]
        n173 = call-poly <vilib>:"Linear Fit Intervals.vi"("Y"=w466, "confidence level"="confidence level horz. fringe", "X"=w467, "slope"=w462, "intercept"=w401) -> ("delta slope"=w434:dbl)  [unwired: 6 in, 4 out]
        n174 = call-poly <vilib>:"Linear Fit Intervals.vi"("Y"=w493, "confidence level"="confidence level vert. fringe", "X"=w492, "slope"=w392, "intercept"=w458) -> ("delta slope"=w488:dbl)  [unwired: 6 in, 4 out]
        n175 = local read "horz intercept value"() -> (w375:dbl[])
        n176 = local read "horz.intercept"() -> (w345:dbl)
        n177 = Bundle(w332, "horz intercept value"=w375) -> (→"horzontal intercept":cluster{dbl[], "horz intercept value":dbl[]})  [unwired: 1 in]
        n178 = Divide(x=w488, y=w392) -> (x/y=w486:dbl)
        n179 = local read "Servo motor Current \nAngle (Degrees) 2"() -> (w316:u8)
        n180 = local read "sample length"() -> (w425:i32)
        n181 = local read "sample length"() -> (w436:i32)
        n182 = local read "Servo motor Current \nAngle (Degrees) 2"() -> (w318:u8)
        n183 = Divide(x=w434, y=w462) -> (x/y=w460:dbl)
        n184 = local read "vrt. slope"() -> (w417:dbl)
        n185 = call <vilib>:"Standard Deviation PtByPt.vi"("x"=w403, "sample length"=w425) -> ("standard deviation"=w481:dbl)  [unwired: 1 in, 2 out]
        "standard deviation" <- w481
        n186 = Multiply(x=w417, y=9.0) -> (x*y=w415:dbl)
        n187 = Multiply(x=w460, y=1000000.0) -> (x*y=w459:dbl)
        n188 = Multiply(x=w486, y=1000000.0) -> (x*y=w485:dbl)
        n189 = Divide(x=1.0, y=w345) -> (x/y=w323:dbl)
        "cm-1" <- w323
        n190 = Multiply(x=w415, y=1e-06) -> (x*y=→"d value":dbl)
        n191 = Format Into String(format string="horz. fringe slope error: %5.2f ppm", w459) -> (resulting string=→"?":string)  [unwired: 2 in, 1 out]
        n192 = Build Array (concatenate)(w502, w403) -> (w475:dbl[])
        "vert inteer" <- w475
        n193 = Bundle(w332, w475) -> (→"Vertical intercept vs real time":cluster{dbl[], dbl[]})  [unwired: 1 in]
        n194 = Format Into String(format string="vert. fringe slope error: %5.2f ppm", w485) -> (resulting string=→"?":string)  [unwired: 2 in, 1 out]
        n195 = call <vilib>:"Standard Deviation PtByPt.vi"("x"=w401, "sample length"=w436) -> ("standard deviation"=w439:dbl)  [unwired: 1 in, 2 out]
        "hor. std dev" <- w439
        n196 = Divide(x=w337, y="minimum OPO") -> (x/y=w338:dbl)
        n197 = Multiply(x=w481, y="calibration factor vert. fringe") -> (x*y=w482:dbl)
        n198 = Divide(x=w337, y="maximum OPO") -> (x/y=w335:dbl)
        "x/y" <- w335
        n199 = Build Array (concatenate)(w393, w392) -> (w390:dbl[])
        n200 = Equal?(x=w316, y=u8 180) -> (x = y?=w314:bool)
        n201 = Format Into String(format string="wavelength sens vert fringe: %5.2f MHz", w482) -> (resulting string=→"?":string)  [unwired: 2 in, 1 out]
        n202 = Divide(x=w342, y="minimum 532") -> (x/y=w343:dbl)
        n203 = Multiply(x=w439, y="calibration factor horz. fringe") -> (x*y=w438:dbl)
        n204 = Equal?(x=w318, y=u8 0) -> (x = y?=w317:bool)
        n205 = Bundle(w332, w390) -> (→"Verticle slope":cluster{dbl[], dbl[]})  [unwired: 1 in]
        n206 = flat-sequence {
          tunnel: [w504] -> w309
          tunnel: w314 -> [w504]
          frame #0 {
            n207 = Wait Until Next ms Multiple(millisecond multiple=u32 1500) -> ()  [unwired: 1 out]
          }
        }
        n208 = Greater?(x=w323, y=w335) -> (0:w371:bool)
        n209 = flat-sequence {
          tunnel: [w506] -> w313
          tunnel: w317 -> [w506]
          frame #0 {
            n210 = Wait Until Next ms Multiple(millisecond multiple=u32 1500) -> ()  [unwired: 1 out]
          }
        }
        n211 = Divide(x=w342, y="maximum 532") -> (x/y=w340:dbl)
        n212 = Less?(x=w323, y=w338) -> (x < y?=w372:bool)
        n213 = Format Into String(format string="wavelength sens horz fri: %5.2f MHz", w438) -> (resulting string=→"?":string)  [unwired: 2 in, 1 out]
        n214 = And(x=w371, y=w372) -> (x .and. y?=w312:bool)
        "OPO data" <- w312
        n215 = Less?(x=w323, y=w343) -> (x < y?=w369:bool)
        n216 = Greater?(x=w323, y=w340) -> (0:w370:bool)
        n217 = And(x=w370, y=w369) -> (x .and. y?=w310:bool)
        "532 data" <- w310
        n218 = And(x=w310, y=w309) -> (x .and. y?=w308:bool)
        n219 = And(x=w312, y=w313) -> (x .and. y?=w311:bool)
        n220 = case shown="True" w311 {
          tunnel: w373 -> [w548 w567]
          tunnel: w323 -> [_ w551]
          tunnel: [w548 w566] -> w374
          tunnel: w361 -> [w546 w557]
          tunnel: w360 -> [w547 w556]
          tunnel: w359 -> [_ w555]
          tunnel: w358 -> [_ w554]
          tunnel: [w547 w553] -> w357
          tunnel: [w546 w552] -> w334
          tunnel: w356 -> [w545 w550]
          tunnel: [w545 w549] -> w355
          frame False {
          }
          frame True {
            n221 = Build Array (concatenate)(w567, w551) -> (w566:dbl[])
            "Waveform Graph 2" <- w566
            n222 = Increment(x=w554) -> (x+1=w558:i32)
            n223 = Quotient & Remainder(x=w554, y=w555) -> (x-y*floor(x/y)=w562:i32)  [unwired: 1 out]
            n224 = Index Array(array=w556, index=w562) -> (element=w564:dbl)
            n225 = Less?(x=w555, y=w558) -> (x < y?=w560:bool)
            n226 = Subtract(x=w550, y=w564) -> (x-y=w563:dbl)
            n227 = Select(t=w555, s=w560, f=w558) -> (s? t:f=w559:i32)
            n228 = Replace Array Subset(array=w556, new element=w551, index=w562) -> (w553:dbl[])
            n229 = Add(x=w551, y=w563) -> (x+y=w549:dbl)
            n230 = Divide(x=w549, y=w559) -> (x/y=w565:dbl)
            "Running average 2" <- w565
            n231 = Wait Until Next ms Multiple(millisecond multiple=u32 100) -> ()  [unwired: 1 out]
            n232 = Build Array (concatenate)(w557, w565) -> (w552:dbl[])
            "Running average OPO data" <- w552
          }
        }
        n233 = case shown="True" w308 {
          tunnel: w368 -> [w525 w543]
          tunnel: w323 -> [_ w535]
          tunnel: [w525 w544] -> w367
          tunnel: w358 -> [_ w534]
          tunnel: w359 -> [_ w533]
          tunnel: w366 -> [w524 w532]
          tunnel: [w524 w531] -> w365
          tunnel: [w523 w530] -> w364
          tunnel: w363 -> [w523 w529]
          tunnel: w362 -> [w522 w528]
          tunnel: [w522 w526] -> w333
          frame False {
          }
          frame True {
            n234 = Build Array (concatenate)(w543, w535) -> (w544:dbl[])
            "Waveform Graph" <- w544
            n235 = Increment(x=w534) -> (x+1=w542:i32)
            n236 = Quotient & Remainder(x=w534, y=w533) -> (x-y*floor(x/y)=w538:i32)  [unwired: 1 out]
            n237 = Index Array(array=w532, index=w538) -> (element=w536:dbl)
            n238 = Less?(x=w533, y=w542) -> (x < y?=w540:bool)
            n239 = Subtract(x=w529, y=w536) -> (x-y=w537:dbl)
            n240 = Select(t=w533, s=w540, f=w542) -> (s? t:f=w541:i32)
            n241 = Replace Array Subset(array=w532, new element=w535, index=w538) -> (w531:dbl[])
            n242 = Add(x=w535, y=w537) -> (x+y=w530:dbl)
            n243 = Divide(x=w530, y=w541) -> (x/y=w527:dbl)
            "Running average" <- w527
            n244 = Build Array (concatenate)(w528, w527) -> (w526:dbl[])
            "Running average 532 data" <- w526
            n245 = Wait Until Next ms Multiple(millisecond multiple=u32 100) -> ()  [unwired: 1 out]
          }
        }
        n246 = Build Array (concatenate)(w329, w323) -> (w321:dbl[])
        n247 = Initialize Array(w323, 5 ("dimension size")) -> (w320:dbl[])
        "initialized array" <- w320
        n248 = flat-sequence {
          frame #0 {
            (unwired) 632.807 ("x")
            (unwired) 802.0
            n249 = local read "observed wavelength"() -> (w578:dbl)
            n250 = local read "wedge spacing"() -> (w582:dbl)
            n251 = local read "vert intercept"() -> (w581:dbl)
            n252 = local read "pixel size (nm)"() -> (w584:dbl)
            n253 = Multiply(x=4.0, y=w582) -> (x*y=w611:dbl)
            n254 = Multiply(x=4.0, y=w581) -> (x*y=w607:dbl)
            n255 = Multiply(x=1000000.0, y=w611) -> (x*y=w610:dbl)
            n256 = Multiply(x=2.0, y=w581) -> (x*y=w596:dbl)
            n257 = Multiply(x=2.0, y=w582) -> (x*y=w601:dbl)
            n258 = Multiply(x="pixel size (nm)", y=w607) -> (x*y=w605:dbl)
            n259 = Multiply(x=w584, y=w596) -> (x*y=w593:dbl)
            n260 = local read "wedge angle (rad)"() -> (w583:dbl)
            n261 = local read "wedge angle (rad)"() -> (w579:dbl)
            n262 = Multiply(x=1000000.0, y=w601) -> (x*y=w597:dbl)
            n263 = Tangent(1:w583) -> (0:w606:dbl)
            n264 = Tangent(1:w579) -> (0:w594:dbl)
            n265 = Multiply(x=w594, y=w593) -> (x*y=w589:dbl)
            n266 = Multiply(x=w606, y=w605) -> (x*y=w604:dbl)
            n267 = Add(x=w597, y=w589) -> (x+y=w588:dbl)
            n268 = Divide(x=w588, y=w578) -> (x/y=w592:dbl)
            n269 = Add(x=w604, y=w610) -> (x+y=w599:dbl)
            n270 = Subtract(x=w592, y=0.5) -> (x-y=w590:dbl)
            n271 = Round To Nearest(number=w590) -> (nearest integer value=w586:dbl)
            n272 = Multiply(x=2.0, y=w586) -> (x*y=w585:dbl)
            n273 = Add(x=w585, y=1.0 ("x")) -> (x+y=w598:dbl)
            n274 = Divide(x=w599, y=w598) -> (x/y=→"second pass wl":dbl)
          }
          frame #1 {
            n275 = local read "thor wedge spacing"() -> (w647:dbl)
            n276 = local read "horz.intercept"() -> (w648:dbl)
            n277 = local read "second pass wl"() -> (w618:dbl)
            n278 = local read "pixel size (nm)"() -> (w646:dbl)
            n279 = local read "pixel size (nm)"() -> (w619:dbl)
            n280 = Multiply(x=4.0, y=w647) -> (x*y=w621:dbl)
            n281 = Multiply(x=4.0, y=w648) -> (x*y=w624:dbl)
            n282 = Multiply(x=1000000.0, y=w621) -> (x*y=w622:dbl)
            n283 = local read "wedge angle of thor wedge"() -> (w617:dbl)
            n284 = Multiply(x=2.0, y=w648) -> (x*y=w634:dbl)
            n285 = Multiply(x=2.0, y=w647) -> (x*y=w629:dbl)
            n286 = Multiply(x=w619, y=w624) -> (x*y=w626:dbl)
            n287 = local read "wedge angle of thor wedge"() -> (w616:dbl)
            n288 = Multiply(x=w646, y=w634) -> (x*y=w637:dbl)
            n289 = Multiply(x=1000000.0, y=w629) -> (x*y=w633:dbl)
            n290 = Tangent(1:w616) -> (0:w625:dbl)
            n291 = Tangent(1:w617) -> (0:w636:dbl)
            n292 = Multiply(x=w636, y=w637) -> (x*y=w641:dbl)
            n293 = Multiply(x=w625, y=w626) -> (x*y=w627:dbl)
            n294 = Add(x=w633, y=w641) -> (x+y=w642:dbl)
            n295 = Divide(x=w642, y=w618) -> (x/y=w638:dbl)
            n296 = Add(x=w627, y=w622) -> (x+y=w631:dbl)
            n297 = Subtract(x=w638, y=0.5) -> (x-y=w640:dbl)
            n298 = Round To Nearest(number=w640) -> (nearest integer value=w644:dbl)
            n299 = Multiply(x=2.0, y=w644) -> (x*y=w645:dbl)
            n300 = Add(x=w645, y=1.0 ("x")) -> (x+y=w632:dbl)
            n301 = Divide(x=w631, y=w632) -> (x/y=→"second pass wl 2":dbl)
          }
        }
        n302 = Array Subset(array=w320, index=5, length=5) -> (w326:dbl[])
        n303 = for {
          N: 2 -> [w508]
          tunnel: [w507] -> w325
          i -> [w509]
          n304 = Equal?(x=w508, y=w509) -> (x = y?=w507:bool)
        }
        n305 = case shown="True" w325 {
          tunnel: w326 -> [_ w510]
          frame False {
          }
          frame True {
            "subarray 2" <- w510
          }
        }
        n306 = case shown="True" "Feedback ON" {
          tunnel: w353 -> [_ w516]
          tunnel: w352 -> [_ w512]
          frame False {
          }
          frame True {
            n307 = local read "Process value"() -> (w519:dbl)
            n308 = call-poly <vilib>:"PID.vi"("output range"="output range", "dt (s)"=0.01, "PID gains"="PID gains", "process variable"=w519, "setpoint"="setpoint") -> ("output"=w518:dbl)  [unwired: 5 in, 1 out]
            "output" <- w518
            n309 = Multiply(x=w512, y="Feedback sign") -> (x*y=w514:i32)
            n310 = Add(x=w518, y=w514) -> (x+y=w511:dbl)
            "Output (V)" <- w511
            n311 = call "RIGOL_power_supply(SubVI).vi"("voltage_in 3"=w511, "VISA Refnum in"=w516) -> ()  [unwired: 8 in, 2 out]
          }
        }
        n312 = Subtract(x=w333, y=w334) -> (x-y=w307:dbl[])
        n313 = Absolute Value(x=w307) -> (abs(x)=w306:dbl[])
        "OPO-532" <- w306
        n314 = Bundle(w332, w306) -> (→"OPO-532":cluster{dbl[], dbl[]})  [unwired: 1 in]
        n315 = Array Size(array=w306) -> (size(s)=w351:i32)
        n316 = Decrement(x=w351) -> (x-1=w350:i32)
        n317 = Index Array(array=w306, index=w350) -> (element=→"Process value":dbl)
        "Array 5" <- w332
      }
    }
    "loop_counter" <- w144
  }
  "Array" <- w61
  n318 = Tick Count (ms)() -> (millisecond timer value=→"initial time":u32)
  n319 = call <vilib>:"Close.vi"("Arduino Resource"=w24, "error in"=w23) -> ()  [unwired: 13 in, 1 out]
  n320 = local write "initial array vert"(ext[] array[1280 elements] ("initial array vert")) -> ()
  n321 = local write "initial array vert.  fringe"(ext[] array[640 elements] ("initial array vert.  fringe")) -> ()
  n322 = local write "initial array vert.  fringe"(ext[] array[1280 elements] ("initial array")) -> ()
  n323 = local write "initial array horz"(ext[] array[1280 elements] ("initial array 2")) -> ()
  n324 = local write "initial array vert"(ext[] array[960 elements] ("initial array vert")) -> ()
  n325 = local write "initial array vert.  fringe"(ext[] array[1280 elements] ("initial array")) -> ()
  n326 = local write "initial array horz"(ext[] array[1280 elements] ("initial array 2")) -> ()
  n327 = call <vilib>:"IMAQdx Close Camera.vi"("Session In"=w72) -> ("error out"=w43:errorcluster)  [unwired: 10 in]
  n328 = Build Array(w48, w47, w41, w46) -> (w45:dbl[][])
  n329 = Transpose 2D Array(2D array=w45) -> (transposed array=w44:dbl[][])
  n330 = call-poly <vilib>:"Write Delimited Spreadsheet.vi"("format (%.3f)"="%.5f", "2D data"=w44, "append to file? (new file:F)"=FALSE ("append to file? (F)"), "error in (no error)"=w43) -> ("error out"=→"error out 2":errorcluster)  [unwired: 10 in, 1 out]
  "initial array horz" <- ext[] array[960 elements] ("initial array horz")
  "initial array vert" <- ext[] array[1280 elements] ("initial array vert")
